vi "Update Parameters.vi"(8 "error in (no error)":errorcluster, 11 "Ruby Spectra in":refnum<class "Ruby Spectra.lvclass">) -> (0 "error out":errorcluster, 3 "Ruby Spectra out":refnum<class "Ruby Spectra.lvclass">)   [LabVIEW 2016, in "Ruby Spectra.lvclass"]
uses:
  Ruby Spectra.lvclass
  C:/GitHub/LabActor/Recorders/Spectrometer/Spectrometer.lvclass
  NHMFL_Core/Libraries/Instruments/Spectrometer Driver/Spectrometer Driver.lvclass/Spectrometer Driver.ctl
  NHMFL_Core/Libraries/Instruments/Ocean Optics/Ocean Optics Driver/Ocean optics configuration.ctl
  NHMFL_Core/Libraries/Utilities/Fit/Multi-peak Parameters.ctl
  NHMFL_Core/Libraries/Utilities/Fit/Peak Parameters.ctl
  Ruby Spectra.lvclass/Ruby Spectra.ctl
  NHMFL_Core/Libraries/Instruments/Spectrometer Driver/Read Peaks.vi
  NHMFL_Core/Libraries/Instruments/Spectrometer Driver/Spectrometer Driver.lvclass
  C:/GitHub/NHMFL_Core/Libraries/Instruments/Instrument Driver/Instrument Driver.lvclass
  Spectrometer/Read Spectrometer Driver.lvclass.vi
  Read Rubi spectra configuration.vi
  NHMFL_Core/Libraries/Instruments/Instrument Driver/Read User configuration.vi
  NHMFL_Core/Libraries/Instruments/Instrument Driver/Write User configuration.vi
  Spectrometer/Write Spectrometer Driver.lvclass.vi
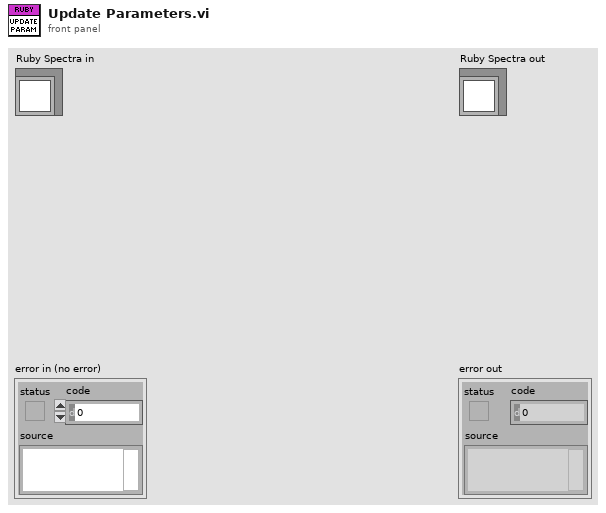
[diagram p1: front panel]
types:
  T1 = typedef "Ruby Spectra.lvclass/Ocean optics configuration.ctl" = cluster{"Integration time":dbl, "Fit parameters":T2, "Fit":bool, "Auto-update params":bool, "Save spectra":bool, "Reference wavelengh":dbl, "Background":path}
  T2 = typedef "Multi-peak Parameters.ctl" = cluster{"Function":enum16{"Gauss", "Lorentz"}, "Window width":dbl, "Initial guess":T3}
  T3 = typedef "Peak Parameters.ctl" = cluster{"Amplitude":dbl, "Center":dbl, "Width":dbl}
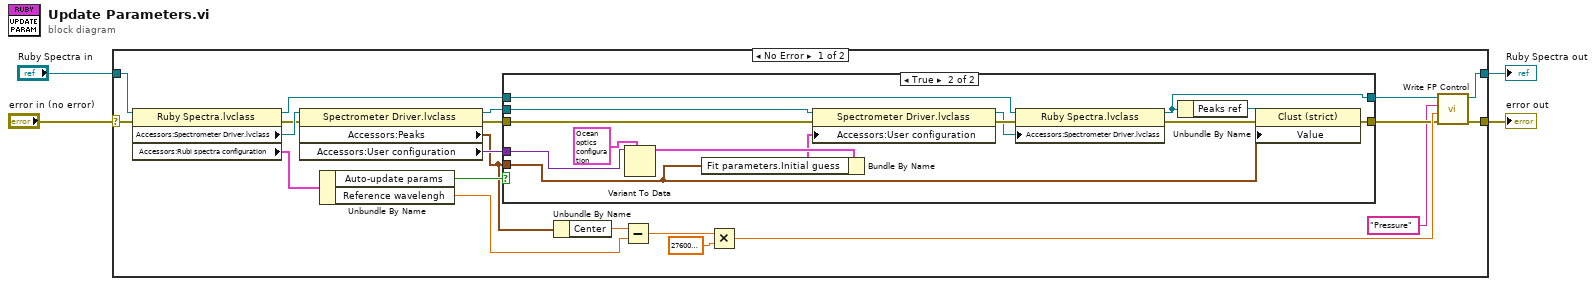
[diagram p0: block diagram]
diagram:
  n1 = case shown="No Error" "error in (no error)" {
    selector: "error in (no error)" -> [w25 w43]
    tunnel: [w6 w43] -> w3
    tunnel: [w9 w42] -> w1
    tunnel: "Ruby Spectra in" -> [w24 w42]
    frame No Error {
      n2 = property class="Ruby Spectra.lvclass"(reference=w24, error in=w25) -> (reference out=w21:refnum<class "Ruby Spectra.lvclass">, error out=w22:errorcluster, "Accessors:Spectrometer Driver.lvclass"=w23:refnum<class "Spectrometer Driver.lvclass">, "Accessors:Rubi spectra configuration"=w20:T1)
      n3 = property class="Spectrometer Driver.lvclass"(reference=w23, error in=w22) -> (reference out=w18:refnum<class "Spectrometer Driver.lvclass">, error out=w17:errorcluster, "Accessors:Peaks"=w15:T3, "Accessors:User configuration"=w19:variant)
      n4 = Unbundle By Name(w20) -> ("Auto-update params"=w16:bool, "Reference wavelengh"=w14:dbl)
      n5 = case shown="True" w16 {
        tunnel: [w26 w40] -> w7
        tunnel: w19 -> [_ w39]
        tunnel: w15 -> [_ w36]
        tunnel: w18 -> [_ w35]
        tunnel: w17 -> [w26 w33]
        tunnel: w21 -> [w27 w30]
        tunnel: [w27 w29] -> w10
        frame False {
        }
        frame True {
          n6 = Variant To Data(type=T1 {"Integration time"=0.5, "Fit parameters"={"Function"=enum."Gauss", "Window width"=0.0, "Initial guess"={"Amplitude"=1000.0, "Center"=694.3, "Width"=0.4}}, "Fit"=TRUE, "Auto-update params"=FALSE, "Save spectra"=FALSE, "Reference wavelengh"=694.123, "Background"=path ""} ("Rubi spectra configuration"), Variant=w39) -> (data=w37:T1)  [unwired: 1 in, 1 out]
          n7 = Bundle By Name(cluster=w37, "Fit parameters.Initial guess"=w36) -> (w34:T1)
          n8 = property class="Spectrometer Driver.lvclass"(reference=w35, error in=w33, "Accessors:User configuration"=w34) -> (reference out=w28:refnum<class "Spectrometer Driver.lvclass">, error out=w32:errorcluster)
          n9 = property class="Ruby Spectra.lvclass"(reference=w30, error in=w32, "Accessors:Spectrometer Driver.lvclass"=w28) -> (reference out=w29:refnum<class "Ruby Spectra.lvclass">, error out=w31:errorcluster)
          n10 = Unbundle By Name(w29) -> ("Peaks ref"=w41:refnum<vi>)
          n11 = property class="Clust (strict)"(reference=w41, error in=w31, "Value"=w36) -> (error out=w40:errorcluster)  [unwired: 1 out]
        }
      }
      n12 = Unbundle By Name(w15) -> ("Center"=w13:dbl)
      n13 = Subtract(x=w13, y=w14) -> (x-y=w11:dbl)
      n14 = Multiply(x=w11, y=2760000000.0) -> (x*y=w8:dbl)
      n15 = call-dynamic "Write FP Control.vi"("error in (no error)"=w7, "Control Value"=w8, "Control Name"="Pressure", "Measure Object in"=w10) -> ("error out"=w6:errorcluster, "Measure Object out"=w9:refnum<class "Ruby Spectra.lvclass">)  [unwired: 6 in]
    }
    frame Error {
    }
  }
  "error out" <- w3
  "Ruby Spectra out" <- w1
